vi "pico.vi"() -> ()   [LabVIEW 2019]
uses:
  Instance           1 15Saved   usbtc08 .vi
  usbtc08.dll
panel:
  out "Min Interval (ms)":i32
  in  "Mains Frequency":i16(ring) items=["50 Hz", "60 Hz"]
  out "?":dynamicdata(graph)
  in  "?":bool
  in  "Ch # 8":bool
  in  "Type # 8":i16(ring)=107 items=["B"=98, "E"=101, "J"=106, "K"=107, "N"=110, "R"=114, "S"=115, "T"=116, "Voltage"=120]
  in  "Ch # 7":bool
  in  "Type # 7":i16(ring)=107 items=["B"=98, "E"=101, "J"=106, "K"=107, "N"=110, "R"=114, "S"=115, "T"=116, "Voltage"=120]
  in  "Ch # 6":bool
  in  "Type # 6":i16(ring)=107 items=["B"=98, "E"=101, "J"=106, "K"=107, "N"=110, "R"=114, "S"=115, "T"=116, "Voltage"=120]
  in  "Ch # 5":bool
  in  "Type # 5":i16(ring)=107 items=["B"=98, "E"=101, "J"=106, "K"=107, "N"=110, "R"=114, "S"=115, "T"=116, "Voltage"=120]
  in  "Ch # 4":bool
  in  "Type # 4":i16(ring)=107 items=["B"=98, "E"=101, "J"=106, "K"=107, "N"=110, "R"=114, "S"=115, "T"=116, "Voltage"=120]
  in  "Ch # 3":bool
  in  "Type # 3":i16(ring)=107 items=["B"=98, "E"=101, "J"=106, "K"=107, "N"=110, "R"=114, "S"=115, "T"=116, "Voltage"=120]
  in  "Ch# 2":bool=TRUE
  in  "Type # 2":i16(ring)=107 items=["B"=98, "E"=101, "J"=106, "K"=107, "N"=110, "R"=114, "S"=115, "T"=116, "Voltage"=120]
  in  "Ch# 1":bool=TRUE
  in  "Type # 1":i16(ring)=107 items=["B"=98, "E"=101, "J"=106, "K"=107, "N"=110, "R"=114, "S"=115, "T"=116, "Voltage"=120]
  in  "Units":enum16{"C°", "F°", "K°", "R°"}(ring)
  in  "stop":bool
  out "Handle":i16
  # "Display updated every 2 seconds"
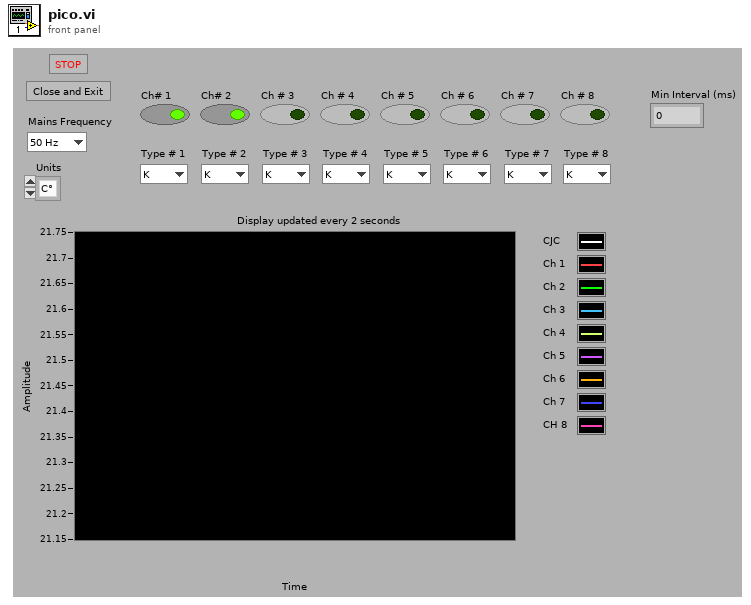
[diagram p1: front panel]
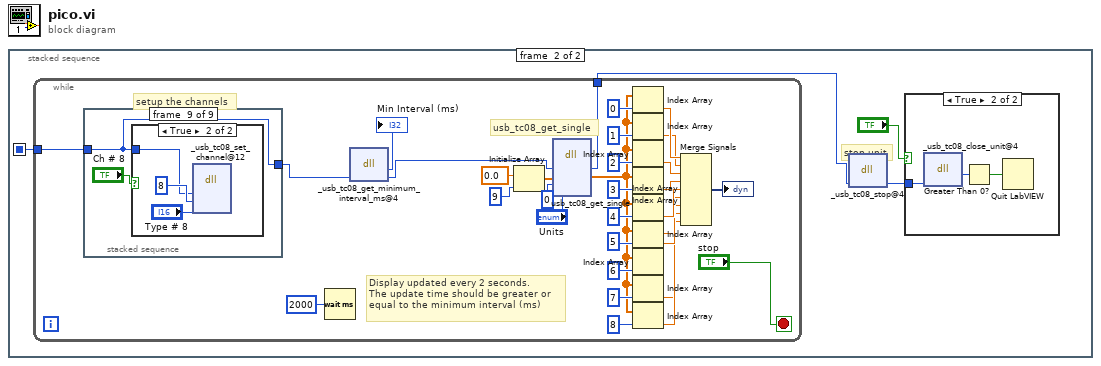
[diagram p0: block diagram]
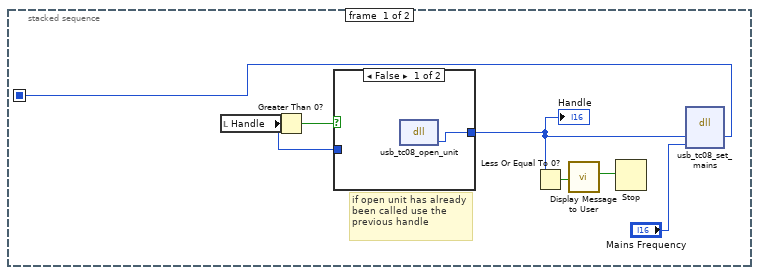
[diagram p2: hidden frame]
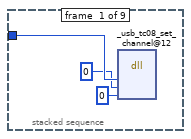
[diagram p4: hidden frame]
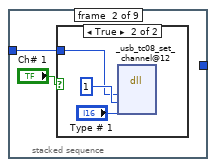
[diagram p5: hidden frame]
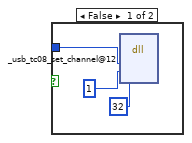
[diagram p6: hidden frame]
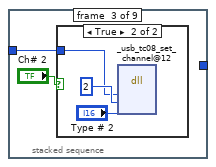
[diagram p7: hidden frame]
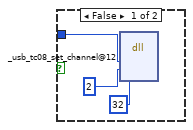
[diagram p8: hidden frame]
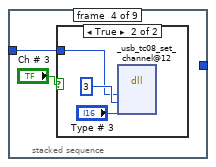
[diagram p9: hidden frame]
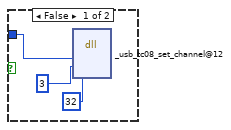
[diagram p10: hidden frame]
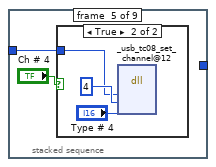
[diagram p11: hidden frame]
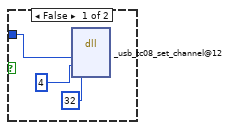
[diagram p12: hidden frame]
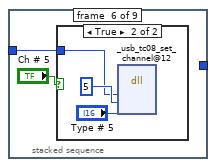
[diagram p13: hidden frame]
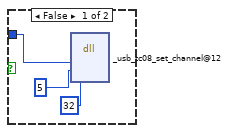
[diagram p14: hidden frame]
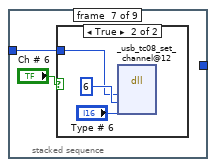
[diagram p15: hidden frame]
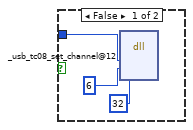
[diagram p16: hidden frame]
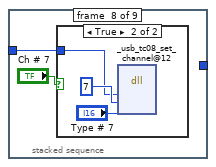
[diagram p17: hidden frame]
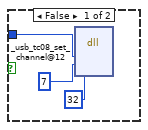
[diagram p18: hidden frame]
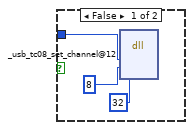
[diagram p19: hidden frame]
diagram:
  n1 = stacked-sequence {
    seq-local: [w5 _] -> [_ w13]
    frame #0 {
      # "if open unit has already been called use the previous handle"
      n2 = local read "Handle"() -> (w6:i16)
      n3 = Greater Than 0?(x=w6) -> (x > 0?=w7:bool)
      n4 = case shown="False" w7 {
        tunnel: [w8 w9] -> w4
        tunnel: w6 -> [_ w9]
        frame False {
          n5 = dll-call lib="usbtc08.dll" fn="usb_tc08_open_unit" label="OpenUnit"() -> ("Handle"=w8:i16)  [unwired: 3 in, 2 out]
        }
        frame True {
        }
      }
      "Handle" <- w4
      n6 = Less Or Equal To 0?(x=w4) -> (x <= 0?=w3:bool)
      n7 = call "Display Message to User"("Enable"=w3) -> ("OK"=w2:bool)  [unwired: 9 in, 1 out]
      n8 = Stop(stop? (T)=w2) -> ()
      n9 = dll-call lib="usbtc08.dll" fn="usb_tc08_set_mains" label="Set Mains"("Handle"=w4, "sixtyHertz"="Mains Frequency") -> ("Handle"=w5:i16)  [unwired: 5 in, 2 out]
    }
    frame #1 {
      # "stop unit"
      n10 = while {
        tunnel: w13 -> [w45]
        tunnel: [w20] -> w10
        stop <- "stop" stop-if-true
        # "Display updated every 2 seconds.\nThe update time should be greater or\nequal to the minimum interval (ms)"
        # "usb_tc08_get_single"
        # "setup the channels"
        n11 = stacked-sequence {
          tunnel: w45 -> [w48 w50 w58 w66 w74 w82 w90 w98 w105]
          tunnel: [_ _ _ _ _ _ _ _ w105] -> w16
          frame #0 {
            n12 = dll-call lib="usbtc08.dll" fn="_usb_tc08_set_channel@12"("handle"=w48, "channel"=i16 0, "tc_type"=i8 0) -> ()  [unwired: 7 in, 2 out]
          }
          frame #1 {
            n13 = case shown="True" "Ch# 1" {
              tunnel: w50 -> [w52 w55]
              frame False {
                n14 = dll-call lib="usbtc08.dll" fn="_usb_tc08_set_channel@12"("handle"=w52, "channel"=i16 1, "tc_type"=32) -> ()  [unwired: 7 in, 2 out]
              }
              frame True {
                n15 = dll-call lib="usbtc08.dll" fn="_usb_tc08_set_channel@12"("handle"=w55, "channel"=i16 1, "tc_type"="Type # 1") -> ()  [unwired: 7 in, 2 out]
              }
            }
          }
          frame #2 {
            n16 = case shown="True" "Ch# 2" {
              tunnel: w58 -> [w59 w63]
              frame False {
                n17 = dll-call lib="usbtc08.dll" fn="_usb_tc08_set_channel@12"("handle"=w59, "channel"=i16 2, "tc_type"=32) -> ()  [unwired: 7 in, 2 out]
              }
              frame True {
                n18 = dll-call lib="usbtc08.dll" fn="_usb_tc08_set_channel@12"("handle"=w63, "channel"=i16 2, "tc_type"="Type # 2") -> ()  [unwired: 7 in, 2 out]
              }
            }
          }
          frame #3 {
            n19 = case shown="True" "Ch # 3" {
              tunnel: w66 -> [w67 w71]
              frame False {
                n20 = dll-call lib="usbtc08.dll" fn="_usb_tc08_set_channel@12"("handle"=w67, "channel"=i16 3, "tc_type"=32) -> ()  [unwired: 7 in, 2 out]
              }
              frame True {
                n21 = dll-call lib="usbtc08.dll" fn="_usb_tc08_set_channel@12"("handle"=w71, "channel"=i16 3, "tc_type"="Type # 3") -> ()  [unwired: 7 in, 2 out]
              }
            }
          }
          frame #4 {
            n22 = case shown="True" "Ch # 4" {
              tunnel: w74 -> [w75 w79]
              frame False {
                n23 = dll-call lib="usbtc08.dll" fn="_usb_tc08_set_channel@12"("handle"=w75, "channel"=i16 4, "tc_type"=32) -> ()  [unwired: 7 in, 2 out]
              }
              frame True {
                n24 = dll-call lib="usbtc08.dll" fn="_usb_tc08_set_channel@12"("handle"=w79, "channel"=i16 4, "tc_type"="Type # 4") -> ()  [unwired: 7 in, 2 out]
              }
            }
          }
          frame #5 {
            n25 = case shown="True" "Ch # 5" {
              tunnel: w82 -> [w83 w87]
              frame False {
                n26 = dll-call lib="usbtc08.dll" fn="_usb_tc08_set_channel@12"("handle"=w83, "channel"=i16 5, "tc_type"=32) -> ()  [unwired: 7 in, 2 out]
              }
              frame True {
                n27 = dll-call lib="usbtc08.dll" fn="_usb_tc08_set_channel@12"("handle"=w87, "channel"=i16 5, "tc_type"="Type # 5") -> ()  [unwired: 7 in, 2 out]
              }
            }
          }
          frame #6 {
            n28 = case shown="True" "Ch # 6" {
              tunnel: w90 -> [w91 w95]
              frame False {
                n29 = dll-call lib="usbtc08.dll" fn="_usb_tc08_set_channel@12"("handle"=w91, "channel"=i16 6, "tc_type"=32) -> ()  [unwired: 7 in, 2 out]
              }
              frame True {
                n30 = dll-call lib="usbtc08.dll" fn="_usb_tc08_set_channel@12"("handle"=w95, "channel"=i16 6, "tc_type"="Type # 6") -> ()  [unwired: 7 in, 2 out]
              }
            }
          }
          frame #7 {
            n31 = case shown="True" "Ch # 7" {
              tunnel: w98 -> [w99 w103]
              frame False {
                n32 = dll-call lib="usbtc08.dll" fn="_usb_tc08_set_channel@12"("handle"=w99, "channel"=i16 7, "tc_type"=32) -> ()  [unwired: 7 in, 2 out]
              }
              frame True {
                n33 = dll-call lib="usbtc08.dll" fn="_usb_tc08_set_channel@12"("handle"=w103, "channel"=i16 7, "tc_type"="Type # 7") -> ()  [unwired: 7 in, 2 out]
              }
            }
          }
          frame #8 {
            n34 = case shown="True" "Ch # 8" {
              tunnel: w105 -> [w107 w111]
              frame False {
                n35 = dll-call lib="usbtc08.dll" fn="_usb_tc08_set_channel@12"("handle"=w107, "channel"=i16 8, "tc_type"=32) -> ()  [unwired: 7 in, 2 out]
              }
              frame True {
                n36 = dll-call lib="usbtc08.dll" fn="_usb_tc08_set_channel@12"("handle"=w111, "channel"=i16 8, "tc_type"="Type # 8") -> ()  [unwired: 7 in, 2 out]
              }
            }
          }
        }
        n37 = Wait (ms)(milliseconds to wait=u32 2000) -> ()  [unwired: 1 out]
        n38 = dll-call lib="usbtc08.dll" fn="_usb_tc08_get_minimum_interval_ms@4"("handle"=w16) -> ("Min Interval (ms)"=→"Min Interval (ms)":i32, "handle"=w15:i16)  [unwired: 3 in, 2 out]
        n39 = Initialize Array(sgl 0.0, i16 9) -> (w44:sgl[])
        n40 = dll-call lib="usbtc08.dll" fn="usb_tc08_get_single"("handle"=w15, "temp_buffer"=w44, "overflow"=i16 0, "units"="Units") -> ("handle"=w20:i16, "temp_buffer"=w30:sgl[])  [unwired: 6 in, 2 out]
        n41 = Index Array(array=w30, index=i16 0) -> (element=w29:sgl)
        n42 = Index Array(array=w30, index=i16 1) -> (element=w19:sgl)
        n43 = Index Array(array=w30, index=i16 2) -> (element=w28:sgl)
        n44 = Index Array(array=w30, index=i16 3) -> (element=w27:sgl)
        n45 = Index Array(array=w30, index=4) -> (element=w26:sgl)
        n46 = Index Array(array=w30, index=i16 5) -> (element=w25:sgl)
        n47 = Index Array(array=w30, index=6) -> (element=w24:sgl)
        n48 = Index Array(array=w30, index=i16 7) -> (element=w22:sgl)
        n49 = Index Array(array=w30, index=i16 8) -> (element=w23:sgl)
        n50 = Merge Signals(w29, w19, w28, w27, w26, w25, w24, w22, w23) -> (→"?":dynamicdata)
      }
      n51 = dll-call lib="usbtc08.dll" fn="_usb_tc08_stop@4" ("Close unit")("handle"=w10) -> ("handle"=w12:i16)  [unwired: 4 in, 2 out]
      n52 = case shown="True" "?" {
        tunnel: w12 -> [_ w115]
        frame False {
        }
        frame True {
          n53 = dll-call lib="usbtc08.dll" fn="_usb_tc08_close_unit@4" ("Close unit")("handle"=w115) -> ("return type"=w114:i16)  [unwired: 4 in, 2 out]
          n54 = Greater Than 0?(x=w114) -> (x > 0?=w113:bool)
          n55 = Quit LabVIEW(quit? (T)=w113) -> ()
        }
      }
    }
  }
